vi "Teleop.vi"(10 "Match Info":T1={"Autonomous Elapsed Seconds"=0.0, "TeleOp Elapsed Seconds"=0.0, "Disabled Elapsed Seconds"=0.0, "Visited Autonomous"=FALSE, "Visited TeleOp"=FALSE, "Visited Disabled"=FALSE, "Autonomous Settings"={"Autonomous Style"=enum."Independent", "VI Refnum"=refnum}}, 11 "Call Context":T2) -> ()   [LabVIEW 2018]
doc: "This VI is called for each TeleOp packet received from the DS where the robot is not disabled. It is often used to read from the joysticks and update I/O or to update setpoints for timed control loops. It should complete and return within 20 milliseconds or it may miss DS packets."
uses:
  <vilib>/Rock Robotics/WPI/DriverStation/WPI_DriverStationDerivedRobotMode.ctl
  <vilib>/Rock Robotics/WPI/DriverStation/WPI_DriverStationMatch Info.ctl
  <vilib>/Rock Robotics/WPI/Utilities/WPI_GetSetVariantRefNum.vi
  Robot Global Data.vi
  <vilib>/Rock Robotics/Network Tables/NT Write Boolean Array.vi
  <vilib>/Rock Robotics/Network Tables/NT Write Numeric Array.vi
  <vilib>/Rock Robotics/Network Tables/NT Read Boolean.vi
  <vilib>/Rock Robotics/Network Tables/NT Read Number.vi
  <vilib>/Rock Robotics/Network Tables/NT Write Number.vi
panel:
  out "Sample Slider 0":dbl(slide) scale=0.0..5.0
  out "Sample Boolean 1":bool
  out "Sample Boolean 0":bool
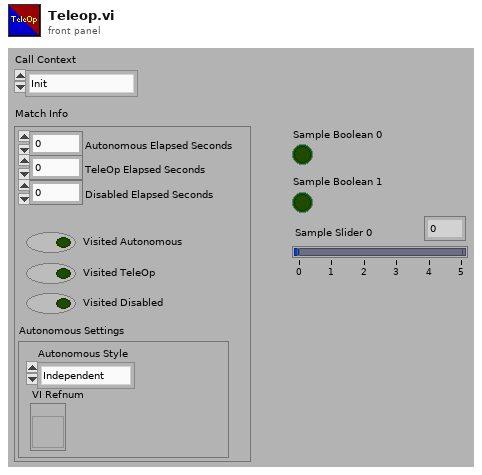
[diagram p1: front panel]
types:
  T1 = typedef "WPI_DriverStationMatch Info.ctl" = cluster{"Autonomous Elapsed Seconds":dbl, "TeleOp Elapsed Seconds":dbl, "Disabled Elapsed Seconds":dbl, "Visited Autonomous":bool, "Visited TeleOp":bool, "Visited Disabled":bool, "Autonomous Settings":cluster{"Autonomous Style":enum16{"Iterative", "Independent"}, "VI Refnum":refnum<vi>}}
  T2 = typedef "WPI_DriverStationDerivedRobotMode.ctl" = enum16{"Init", "Execute", "Stop"}
  T3 = typedef "WPI_JoystickDevRef.ctl" = cluster{"Device":T4}
  T4 = typedef "WPI_JoystickDeviceEnum.ctl" = enum16{"USB 0", "USB 1", "USB 2", "USB 3", "USB 4", "USB 5"}
  T5 = typedef "WPI_RobotDriveDevRef.ctl" = cluster{"DevStatus":errorcluster, "Motors[]":T6[], "Square Inputs":bool, "Max Output":dbl}
  T6 = typedef "WPI_MotorControlDeviceRef.ctl" = cluster{"DeviceStatus":errorcluster, "Type":T7, "PWM":cluster{"PWM Channel":T8, "DeadBand":T9}, "CAN":cluster{"Device Number":u8, "SetOutput VI Ref":variant, "GetOutput VI Ref":variant, "Enable VI Ref":variant, "Disable VI Ref":variant, "Data":variant}, "Invert":bool, "DIO PWM":cluster{"PWM \"Enable\" Channel":T8, "DIOChannel":T10, "PWM Rate":dbl}}
  T7 = typedef "WPI_MotorControlType.ctl" = enum16{"PWM", "CAN", "DIO PWM"}
  T8 = typedef "FPGA_DIOPWMChannel.ctl" = enum8{"PWM 0", "PWM 1", "PWM 2", "PWM 3", "PWM 4", "PWM 5", "PWM 6", "PWM 7", "PWM 8", "PWM 9", "PWM MXP 0", "PWM MXP 1", "PWM MXP 2", "PWM MXP 3", "PWM MXP 4", "PWM MXP 5", "PWM MXP 6", "PWM MXP 7", "PWM MXP 8", "PWM MXP 9", "Invalid"}
  T9 = typedef "WPI_PWMDeadband.ctl" = cluster{"Name":string, "maxPositivePwm":i32, "minPositivePwm":i32, "centerPwm":i32, "maxNegativePwm":i32, "minNegativePwm":i32, "angularRange":u16}
  T10 = typedef "FPGA_DIOChannel.ctl" = enum8{"DIO 0", "DIO 1", "DIO 2", "DIO 3", "DIO 4", "DIO 5", "DIO 6", "DIO 7", "DIO 8", "DIO 9", "DIO MXP 0", "DIO MXP 1", "DIO MXP 2", "DIO MXP 3", "DIO MXP 4", "DIO MXP 5", "DIO MXP 6", "DIO MXP 7", "DIO MXP 8", "DIO MXP 9", "DIO MXP 10", "DIO MXP 11", "DIO MXP 12", "DIO MXP 13", "DIO MXP 14", "DIO MXP 15", "SPI Port CS1", "SPI Port CS2", "SPI Port CS3", "SPI Port MISO", "SPI Port MOSI", "Invalid"}
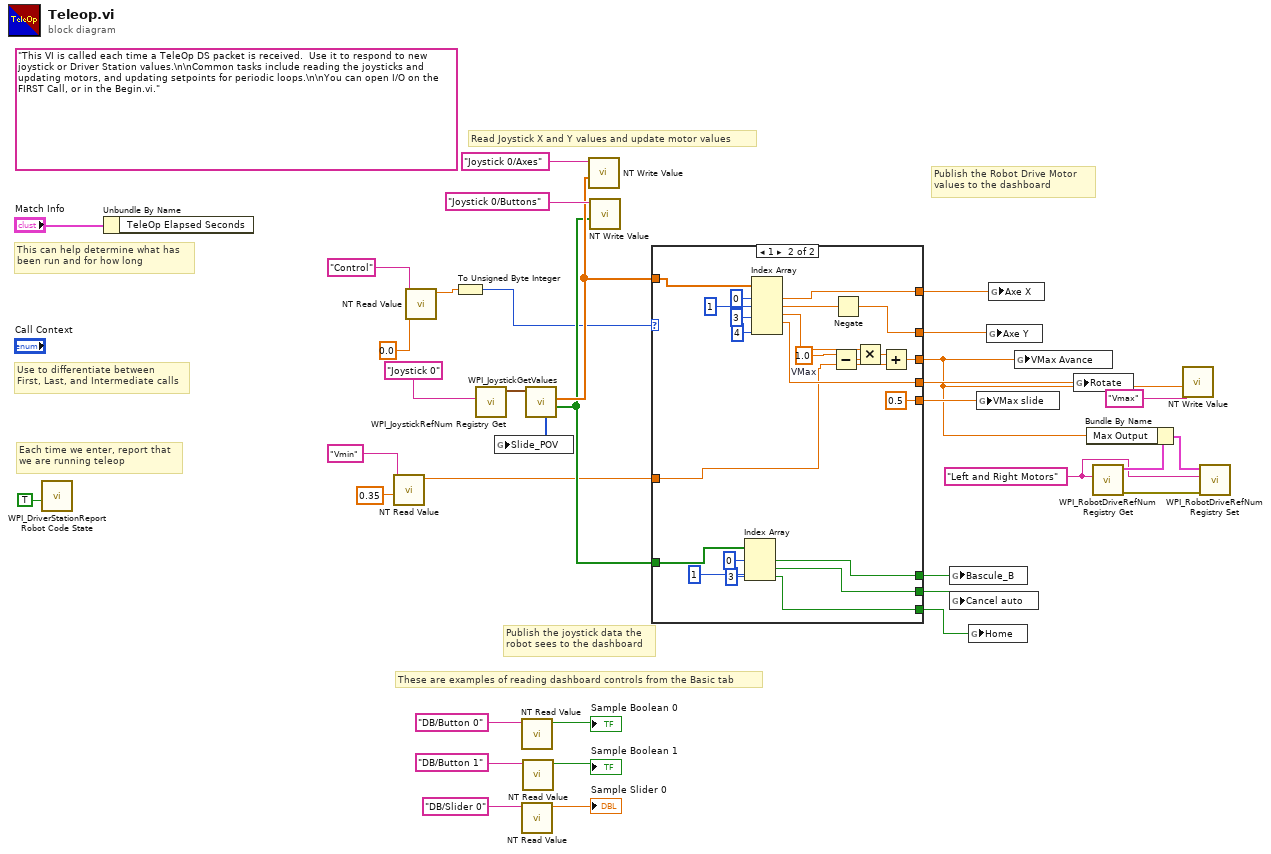
[diagram p0: block diagram]
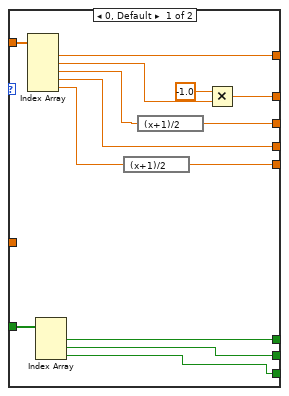
[diagram p2: hidden frame]
diagram:
  w14 = "Left and Right Motors" ("refnum name")
  (unwired) "This VI is called each time a TeleOp DS packet is received.  Use it to respond to new joystick or Driver Station values.\n\nCommon tasks include reading the joysticks and updating motors, and updating setpoints for periodic loops.\n\nYou can open I/O on the FIRST Call, or in the Begin.vi."
  # "These are examples of reading dashboard controls from the Basic tab"
  # "Publish the Robot Drive Motor\nvalues to the dashboard"
  # "Publish the joystick data the\nrobot sees to the dashboard"
  # "Each time we enter, report that\nwe are running teleop"
  # "Use to differentiate between\nFirst, Last, and Intermediate calls"
  # "This can help determine what has\nbeen run and for how long"
  # "Read Joystick X and Y values and update motor values"
  n1 = call <vilib>:"WPI_DriverStationReport Robot Code State.vi"("TeleOp"=TRUE ("Autonomous")) -> ()  [unwired: 10 in, 1 out]
  n2 = Unbundle By Name("Match Info") -> ()  [unwired: 1 out]
  n3 = call-poly <vilib>:"NT Read Value.vi"("Default Value"=0.35, "Name"="Vmin") -> ("Numeric"=w2:dbl)  [unwired: 8 in, 1 out]
  n4 = call-poly <vilib>:"NT Read Value.vi"("Default Value"=0.0, "Name"="Control") -> ("Numeric"=w10:dbl)  [unwired: 8 in, 1 out]
  n5 = To Unsigned Byte Integer(number=w10) -> (unsigned 8bit integer=w9:u8)
  n6 = call <vilib>:"WPI_JoystickRefNum Registry Get.vi"("refnum name"="Joystick 0") -> ("JoystickDevRef"=w33:T3)  [unwired: 1 in, 9 out]
  n7 = call-poly <vilib>:"NT Read Value.vi"("Name"="DB/Button 0" ("refnum name")) -> ("Boolean"=→"Sample Boolean 0":bool)  [unwired: 9 in, 1 out]
  n8 = call-poly <vilib>:"NT Read Value.vi"("Name"="DB/Slider 0" ("refnum name")) -> ("Numeric"=→"Sample Slider 0":dbl)  [unwired: 9 in, 1 out]
  n9 = call-poly <vilib>:"NT Read Value.vi"("Name"="DB/Button 1" ("refnum name")) -> ("Boolean"=→"Sample Boolean 1":bool)  [unwired: 9 in, 1 out]
  n10 = call <vilib>:"WPI_JoystickGetValues.vi"("JoystickDevRef"=w33) -> ("Buttons"=w20:bool[], "Axes"=w29:dbl[], "POVs"=w18:i16[])  [unwired: 6 in, 2 out]
  n11 = global write "Robot Global Data.vi" "Slide_POV"(w18) -> ()
  n12 = call-poly <vilib>:"NT Write Value.vi"("Numeric Array"=w29, "Name"="Joystick 0/Axes") -> ()  [unwired: 9 in, 1 out]
  n13 = call-poly <vilib>:"NT Write Value.vi"("Boolean Array"=w20, "Name"="Joystick 0/Buttons") -> ()  [unwired: 9 in, 1 out]
  n14 = case shown="1" w9 {
    tunnel: w29 -> [w49 w72]
    tunnel: [w48 w71] -> w22
    tunnel: [w47 w56] -> w21
    tunnel: w20 -> [w44 w63]
    tunnel: [w43 w62] -> w19
    tunnel: [w42 w65] -> w17
    tunnel: [w40 w51] -> w4
    tunnel: [w38 0.5 ("upper limit")] -> w12
    tunnel: [w37 w58] -> w7
    tunnel: [w36 w57] -> w6
    tunnel: w2 -> [_ w50]
    frame 0, Default {
      n15 = Index Array(array=w49) -> (element #1=w48:dbl, element #2=w45:dbl, element #3=w41:dbl, element #4=w42:dbl, element #5=w39:dbl)  [unwired: 5 in]
      n16 = Index Array(array=w44) -> (element #1=w43:bool, element #2=w37:bool, element #3=w36:bool)  [unwired: 3 in]
      n17 = expression code="(x+1)/2"(w39) -> (w38:dbl)
      n18 = expression code="(x+1)/2"(w41) -> (w40:dbl)
      n19 = Multiply(x=-1.0, y=w45) -> (x*y=w47:dbl)
    }
    frame 1 {
      w55 = 1.0  # VMax
      n20 = Index Array(array=w63, index #1=0 ("index"), index #2=1 ("index"), index #3=3 ("index")) -> (element #1=w62:bool, element #2=w58:bool, element #3=w57:bool)
      n21 = Index Array(array=w72, index #1=0 ("index"), index #2=1 ("index"), index #3=3 ("index"), index #4=4 ("index")) -> (element #1=w71:dbl, element #2=w70:dbl, element #3=w52:dbl, element #4=w65:dbl)  [unwired: 1 in, 1 out]
      n22 = Subtract(x=w55, y=w50) -> (x-y=w54:dbl)
      n23 = Negate(x=w70) -> (-x=w56:dbl)
      n24 = Multiply(x=w52, y=w54) -> (x*y=w53:dbl)
      n25 = Add(x=w53, y=w50) -> (x+y=w51:dbl)
    }
  }
  n26 = global write "Robot Global Data.vi" "Bascule_B"(w19) -> ()
  n27 = global write "Robot Global Data.vi" "Cancel auto"(w7) -> ()
  n28 = global write "Robot Global Data.vi" "Home"(w6) -> ()
  n29 = global write "Robot Global Data.vi" "VMax slide"(w12) -> ()
  n30 = global write "Robot Global Data.vi" "Axe Y"(w21) -> ()
  n31 = global write "Robot Global Data.vi" "Axe X"(w22) -> ()
  n32 = global write "Robot Global Data.vi" "VMax Avance"(w4) -> ()
  n33 = global write "Robot Global Data.vi" "Rotate"(w17) -> ()
  n34 = call <vilib>:"WPI_RobotDriveRefNum Registry Get.vi"("refnum name"=w14) -> ("error out"=w13:errorcluster, "RobotDriveDevRef"=w16:T5)  [unwired: 1 in, 8 out]
  n35 = Bundle By Name(cluster=w16, "Max Output"=w4) -> (w15:T5)
  n36 = call-poly <vilib>:"NT Write Value.vi"("Numeric"=w4, "Name"="Vmax") -> ()  [unwired: 9 in, 1 out]
  n37 = call <vilib>:"WPI_RobotDriveRefNum Registry Set.vi"("error in (no error)"=w13, "refnum name"=w14, "RobotDriveDevRef"=w15) -> ()  [unwired: 7 in, 2 out]
